vi "interpret data.vi"(0 "data":T1[](array[typedef]) {"time (global)" format="%<%H:%M:%S\n%d/%m/%Y>T"}, 11 "anzahl sources":i32) -> (4 "source data out":dbl[][](array[numeric]), 8 "calibration data out":dbl[][](array[numeric]), 15 "log":T1[](array[typedef]) {"time (global)" format="%<%H:%M:%S\n%d/%m/%Y>T"})   [LabVIEW 2010, in "Licor-Steuerung.lvlib"]
uses:
  Licor-Steuerung.lvlib
  LicorLI7000/conventions/output line.ctl
  LicorLI7000/LicorLI7000.lvlib
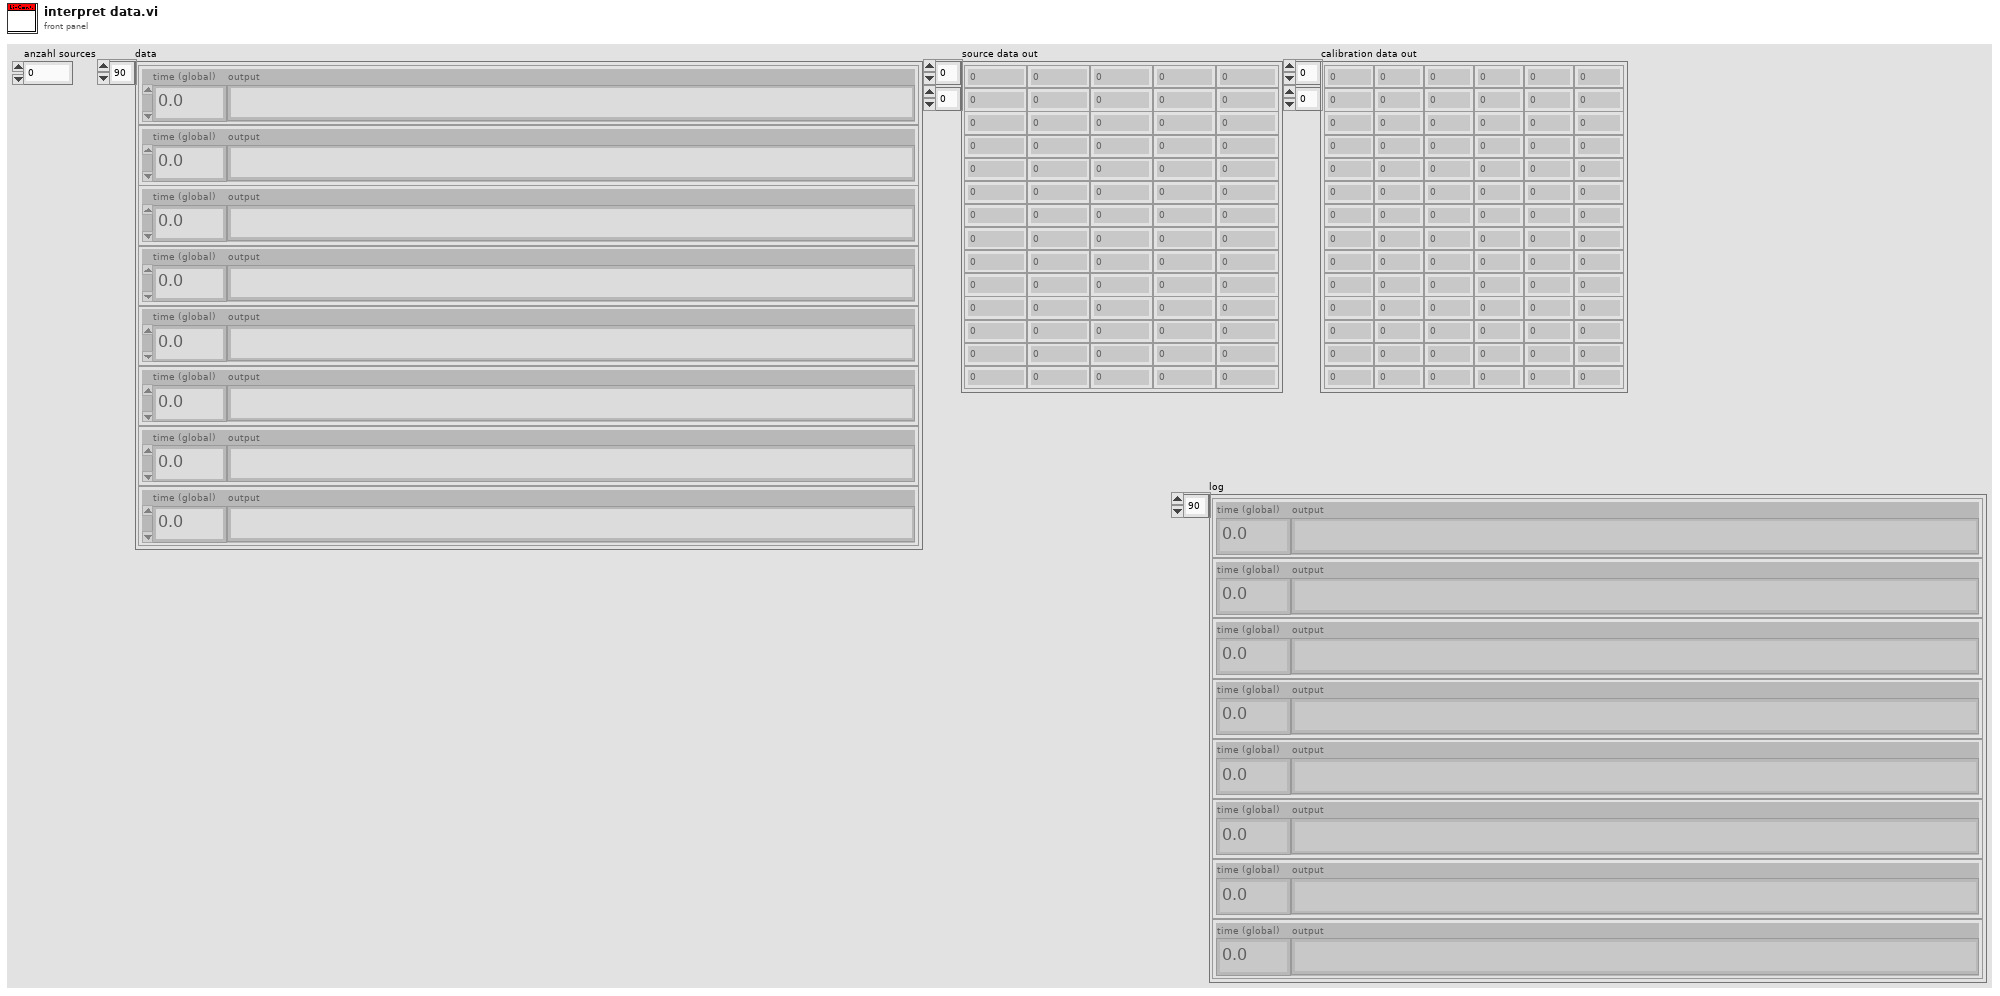
[diagram p1: front panel]
types:
  T1 = typedef "LicorLI7000.lvlib/output line.ctl" = cluster{"time (global)":dbl, "output":string}
  T2 = typedef "LicorLI7000.lvlib/datentyp.ctl" = enum16{"source", "calibration", "LOG"}
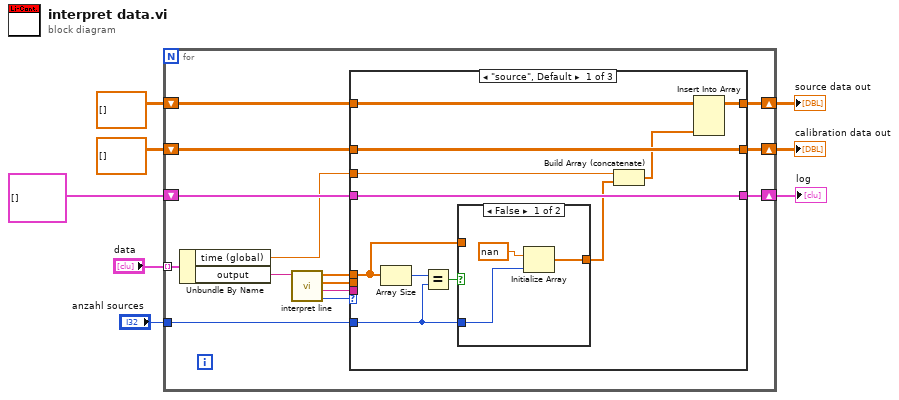
[diagram p0: block diagram]
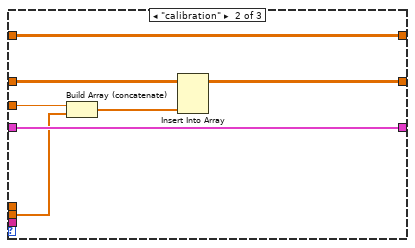
[diagram p3: hidden frame]
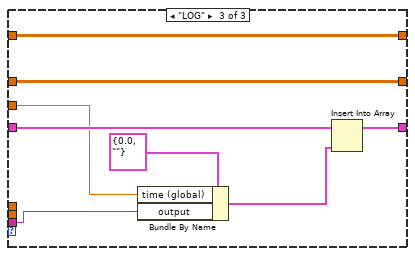
[diagram p4: hidden frame]
diagram:
  n1 = for {
    tunnel: "data" -> [w12] mode=indexing
    shift-right: [w15] -> w1
    shift-left: T1[] [] ("log") -> [w17]
    shift-right: [w13] -> w5
    shift-left: dbl[][] [] -> [w14]
    shift-right: [w22] -> w8
    shift-left: dbl[][] [] -> [w21]
    tunnel: "anzahl sources" -> [w10]
    n2 = Unbundle By Name(w12) -> ("time (global)"=w9:dbl, "output"=w11:string)
    n3 = call "interpret line.vi"("line"=w11) -> ("datentyp"=w20:T2, "LOG"=w16:string, "calibration data out"=w18:dbl[], "source data out"=w19:dbl[])  [unwired: 4 in]
    n4 = case shown="\"source\", Default" w20 {
      tunnel: [w32 w42 w50] -> w22
      tunnel: w21 -> [w33 w42 w50]
      tunnel: w19 -> [w27 _ _]
      tunnel: w18 -> [_ w39 _]
      tunnel: w17 -> [w30 w41 w52]
      tunnel: w16 -> [_ _ w46]
      tunnel: [w30 w41 w51] -> w15
      tunnel: w14 -> [w31 w44 w49]
      tunnel: [w31 w43 w49] -> w13
      tunnel: w10 -> [w23 _ _]
      tunnel: w9 -> [w25 w40 w47]
      frame "source", Default {
        n5 = Array Size(array=w27) -> (size(s)=w29:i32)
        n6 = Equal?(x=w29, y=w23) -> (x = y?=w28:bool)
        n7 = case shown="False" w28 {
          tunnel: w27 -> [_ w37]
          tunnel: [w34 w37] -> w26
          tunnel: w23 -> [w35 _]
          frame False {
            n8 = Initialize Array(nan ("Element"), w35) -> (w34:dbl[])
          }
          frame True {
          }
        }
        n9 = Build Array (concatenate)(w25, w26) -> (w24:dbl[])
        n10 = Insert Into Array(array=w33, new element=w24) -> (w32:dbl[][])  [unwired: 2 in]
      }
      frame "calibration" {
        n11 = Build Array (concatenate)(w40, w39) -> (w38:dbl[])
        n12 = Insert Into Array(array=w44, new element=w38) -> (w43:dbl[][])  [unwired: 2 in]
      }
      frame "LOG" {
        n13 = Bundle By Name(cluster=T1 {"time (global)"=0.0, "output"=""} ("output line"), "time (global)"=w47, "output"=w46) -> (w45:T1)
        n14 = Insert Into Array(array=w52, new element=w45) -> (w51:T1[])  [unwired: 1 in]
      }
    }
  }
  "calibration data out" <- w5
  "source data out" <- w8
  "log" <- w1
